vi "SetIntakeState.vi"(11 "States Enum":T1) -> ()   [LabVIEW 2017]
uses:
  Implementation/Intake Operations.ctl
panel:
  # "input state enum"
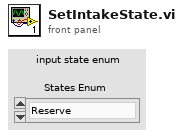
[diagram p1: front panel]
types:
  T1 = typedef "Intake Operations.ctl" = enum16{"Reserve", "Read Current", "setSetpoint", "feed", "spit"}
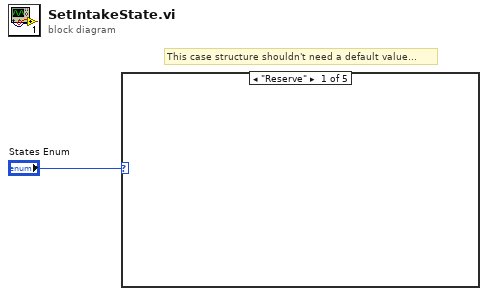
[diagram p0: block diagram]
diagram:
  # "This case structure shouldn't need a default value..."
  n1 = case shown="\"Reserve\"" "States Enum" {
    frame "Reserve" {
    }
    frame "Read Current" {
    }
    frame "setSetpoint" {
    }
    frame "feed" {
    }
    frame "spit" {
    }
  }
